vi "FuzzyDraw.vi"(11 "fuzzy system in":T1 {"user MF interpolating polynomials"."coa_x(y) coeff" format="%.4g"; "user MF interpolating polynomials"."Area(y) coeff" format="%.4g"; "user MF interpolating polynomials"."X(y) coeff" format="%.4g"; "user MF interpolating polynomials"."Y(x) coeff" format="%.4g"; "user MF interpolating polynomials"."Y" format="%.4g"; "user MF interpolating polynomials"."X" format="%.4g"; "defuzzification method" items=["Center of Area", "Modified Center of Area", "Center of Sums", "Center of Maximum", "Mean of Maximum"]; "rules"."consequents"."Var Index" min=0; "rules"."consequents"."Cond" items=["=", "!="]; "rules"."consequents"."MF Index" min=0; "rules"."antecedents"."Var Index" min=0; "rules"."antecedents"."Cond" items=["=", "!="]; "rules"."antecedents"."MF Index" min=0; "rules"."consequent implication" items=["Minimum", "Product"]; "rules"."antecedent connective" items=["AND (Minimum)", "AND (Product)", "OR (Maximum)", "OR (Probabilistic)"]; "output variables"."MFs"."shape" items=["Triangle", "Trapezoid", "Singleton", "Sigmoid", "Gaussian", "User-Defined"]; "input variables"."MFs"."shape" items=["Triangle", "Trapezoid", "Singleton", "Sigmoid", "Gaussian", "User-Defined"]}) -> (1 "Output":cluster{cluster{"Xi":dbl, "Yi":dbl}[]}[](graph), 2 "Error":cluster{cluster{"Xi":dbl, "Yi":dbl}[]}[](graph), 3 "Temperature":cluster{cluster{"Xi":dbl, "Yi":dbl}[]}[](graph))   [LabVIEW 2022 SP3]
uses:
  <vilib>/addons/Fuzzy Logic/TypeDefs/FL System.ctl
  <vilib>/addons/Fuzzy Logic/TypeDefs/FL Variable.ctl
  <vilib>/addons/Fuzzy Logic/TypeDefs/FL Membership Function.ctl
  <vilib>/addons/Fuzzy Logic/TypeDefs/FL Membership Function Shape.ctl
  <vilib>/addons/Fuzzy Logic/TypeDefs/FL Rule.ctl
  <vilib>/addons/Fuzzy Logic/TypeDefs/FL Antecedent.ctl
  <vilib>/addons/Fuzzy Logic/TypeDefs/FL Modifier.ctl
  <vilib>/addons/Fuzzy Logic/TypeDefs/FL Antecedent Connective.ctl
  <vilib>/addons/Fuzzy Logic/TypeDefs/FL Consequent.ctl
  <vilib>/addons/Fuzzy Logic/TypeDefs/FL Consequent Implication.ctl
  <vilib>/addons/Fuzzy Logic/TypeDefs/FL Defuzzification.ctl
  <vilib>/addons/Fuzzy Logic/TypeDefs/FL Interpolating polynomials.ctl
  <vilib>/addons/Fuzzy Logic/TypeDefs/FL Input_Output.ctl
  <vilib>/addons/Fuzzy Logic/NI_Fuzzy_Logic_API.lvlib
panel:
  # "IF"
  # "THEN"
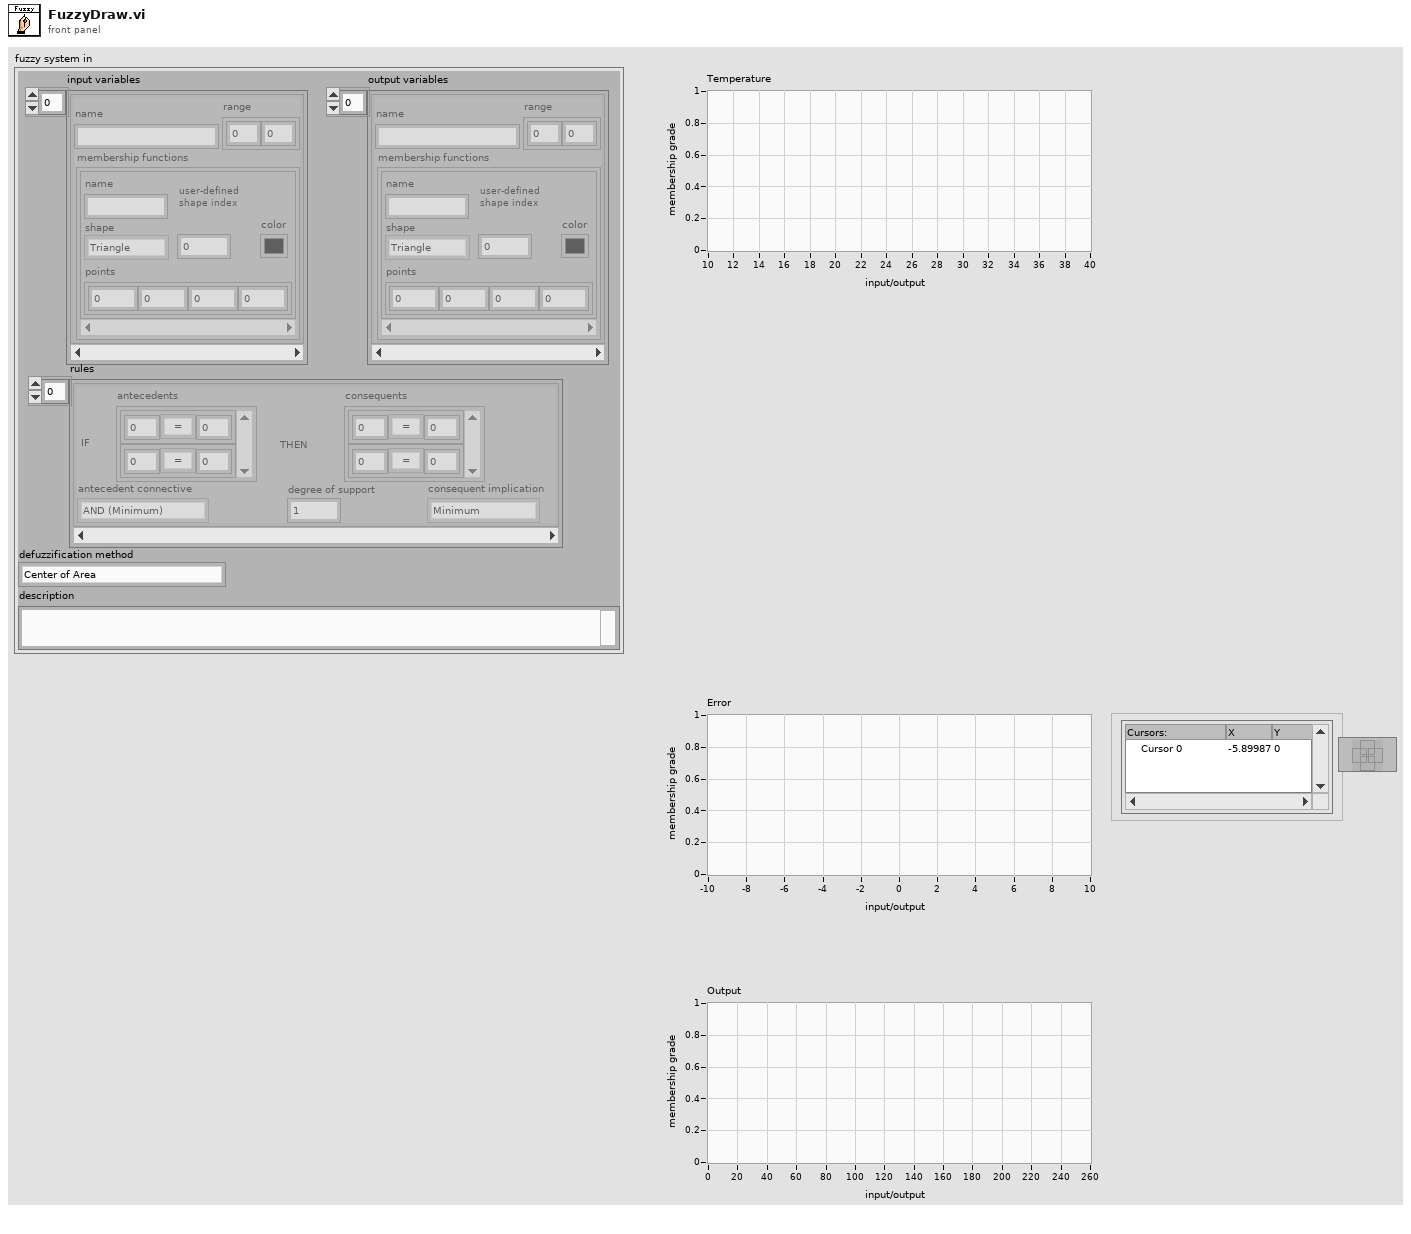
[diagram p1: front panel]
types:
  T1 = typedef "NI_Fuzzy_Logic_API.lvlib/FL System.ctl" = cluster{"input variables":T2[], "output variables":T2[], "rules":T5[], "defuzzification method":T11, "description":string, "user MF interpolating polynomials":T12[]}
  T2 = typedef "NI_Fuzzy_Logic_API.lvlib/FL Variable.ctl" = cluster{"name":string, "range":dbl[], "MFs":T3[]}
  T3 = typedef "NI_Fuzzy_Logic_API.lvlib/FL Membership Function.ctl" = cluster{"name":string, "shape":T4, "points":dbl[], "color":u32, "user-defined shape index":i32}
  T4 = typedef "NI_Fuzzy_Logic_API.lvlib/FL Membership Function Shape.ctl" = u16
  T5 = typedef "NI_Fuzzy_Logic_API.lvlib/FL Rule.ctl" = cluster{"antecedents":T6[], "antecedent connective":T8, "consequents":T9[], "consequent implication":T10, "degree of support":dbl}
  T6 = typedef "NI_Fuzzy_Logic_API.lvlib/FL Antecedent.ctl" = cluster{"Var Index":i32, "MF Index":i32, "Cond":T7}
  T7 = typedef "NI_Fuzzy_Logic_API.lvlib/FL Modifier.ctl" = u16
  T8 = typedef "NI_Fuzzy_Logic_API.lvlib/FL Antecedent Connective.ctl" = u16
  T9 = typedef "NI_Fuzzy_Logic_API.lvlib/FL Consequent.ctl" = cluster{"Var Index":i32, "MF Index":i32, "Cond":T7}
  T10 = typedef "NI_Fuzzy_Logic_API.lvlib/FL Consequent Implication.ctl" = u16
  T11 = typedef "NI_Fuzzy_Logic_API.lvlib/FL Defuzzification.ctl" = u16
  T12 = typedef "NI_Fuzzy_Logic_API.lvlib/FL Interpolating polynomials.ctl" = cluster{"X":dbl[], "Y":dbl[], "Y(x) coeff":dbl[][], "X(y) coeff":dbl[][], "Area(y) coeff":dbl[][], "coa_x(y) coeff":dbl[][]}
  T13 = typedef "NI_Fuzzy_Logic_API.lvlib/FL Input_Output.ctl" = u16
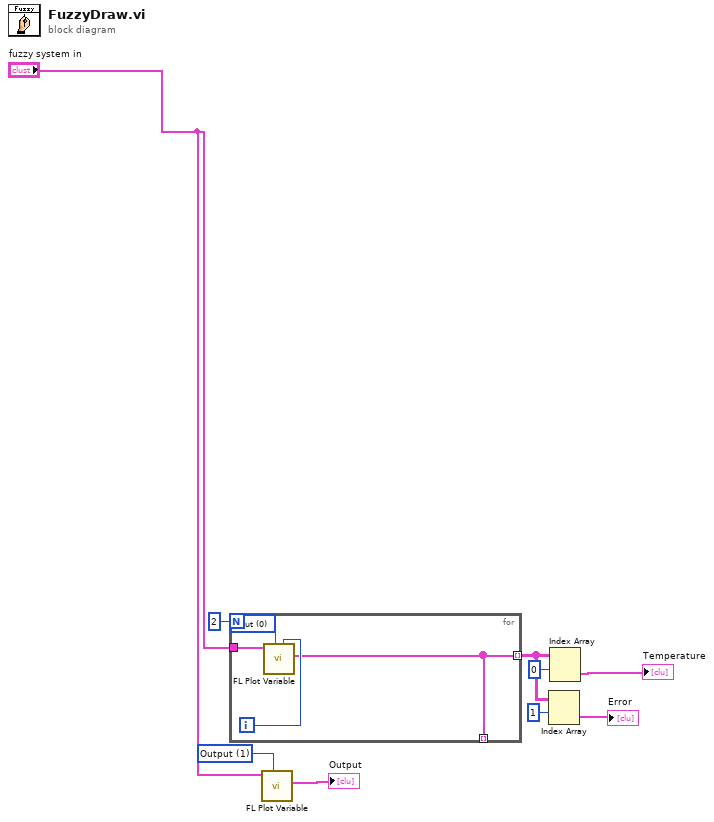
[diagram p0: block diagram]
diagram:
  w1 = T13 1 items=["Input", "Output"] ("input/output")
  n1 = for {
    N: 2 -> [_]
    tunnel: [w10] -> w4 mode=indexing
    tunnel: "fuzzy system in" -> [w11]
    tunnel: [w10] -> _ mode=indexing
    i -> [w12]
    w13 = T13 0 items=["Input", "Output"] ("input/output")
    n2 = call <vilib>:"FL Plot Variable.vi"("variable index"=w12, "input/output"=w13, "fuzzy system in"=w11) -> ("membership functions plot"=w10:cluster{cluster{"Xi":dbl, "Yi":dbl}[]}[])  [unwired: 6 in, 2 out]
  }
  n3 = call <vilib>:"FL Plot Variable.vi"("input/output"=w1, "fuzzy system in"="fuzzy system in") -> ("membership functions plot"=→"Output":cluster{cluster{"Xi":dbl, "Yi":dbl}[]}[])  [unwired: 7 in, 2 out]
  n4 = Index Array(array=w4, index (row)=1) -> (element=→"Error":cluster{cluster{"Xi":dbl, "Yi":dbl}[]}[])  [unwired: 1 in]
  n5 = Index Array(array=w4, index (row)=0) -> (element=→"Temperature":cluster{cluster{"Xi":dbl, "Yi":dbl}[]}[])  [unwired: 1 in]
